vi "IP Connected.vi"(11 "IP Address to Ping":string) -> (3 "Connected":bool)   [LabVIEW 2017]
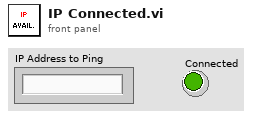
[diagram p1: front panel]
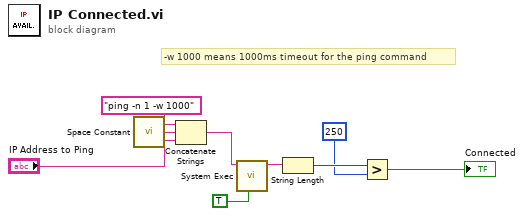
[diagram p0: block diagram]
diagram:
  # "-w 1000 means 1000ms timeout for the ping command"
  n1 = call <vilib>:"Space Constant.vi"() -> ("String"=w8:string)
  n2 = Concatenate Strings("ping -n 1 -w 1000", w8, "IP Address to Ping") -> (w6:string)
  n3 = call <vilib>:"System Exec.vi"("run minimized? (F)"=TRUE, "command line"=w6) -> ("standard output"=w5:string)  [unwired: 6 in, 3 out]
  n4 = String Length(string=w5) -> (length=w4:i32)
  n5 = Greater?(x=w4, y=250) -> (0:→"Connected":bool)
